vi "Task2.vi"() -> ()   [LabVIEW 2021]
uses:
  <vilib>/myRIO/Instrument Drivers/Utilities/Utilities.lvlib
  <vilib>/Platform/TimedLoop/XDataNode/wakeup.ctl
  <vilib>/Platform/TimedLoop/XDataNode/XDNodeRunTimeDep.lvlib
  <vilib>/Platform/TimedLoop/XDataNode/nitl_modes.ctl
  <vilib>/Platform/TimedLoop/XDataNode/timing_clust.ctl
  <vilib>/Platform/TimedLoop/XDataNode/XDataNode.xnode
  <vilib>/myRIO/Instrument Drivers/Onboard IO/AI/AI.lvlib
  <vilib>/myRIO/Common/Instrument Driver Framework/Utilities/typedefs/Analog Scaling Constants.ctl
  <vilib>/myRIO/Common/Instrument Driver Framework/Utilities/typedefs/Analog Scaling Constants List.ctl
  <vilib>/myRIO/Common/Instrument Driver Framework/myRIO v1.0/AI/typedefs/AI Channels Enum.ctl
  <vilib>/myRIO/Common/Instrument Driver Framework/myRIO v1.0/AI/typedefs/AI Channels List.ctl
  <vilib>/myRIO/Common/Instrument Driver Framework/Utilities/typedefs/Generic FPGA Reference.ctl
  <vilib>/myRIO/Common/Instrument Driver Framework/Utilities/typedefs/myRIO v1.0 Reference.ctl
  <vilib>/myRIO/Common/Instrument Driver Framework/Utilities/typedefs/Hardware Version Enum.ctl
  <vilib>/myRIO/Common/Instrument Driver Framework/Utilities/typedefs/myRIO Generic Hardware Reference.ctl
  <vilib>/myRIO/Instrument Drivers/Onboard IO/AI/typedefs/AI Reference.ctl
  <vilib>/userDefined/High Color/nirio_resource_hc.ctl
  <vilib>/myRIO/Common/Instrument Driver Framework/myRIO v1.0/AI/vis/myRIO v1.1 Open AI.vi
  <vilib>/myRIO/Instrument Drivers/Onboard IO/AI/vis/myRIO AI Open.xnode
panel:
  in  "Stop Button":bool
  in  "Tab Control":enum32{"Noise Exposure", "Custom Graphs"}(tab)
  in  "Graph Time Max":dbl=5.0
  in  "Graph Time Min":dbl
  out "Microphone":waveform(dbl)(graph)
  in  "Seconds to Record":dbl=2.0 min=0.0 step=0.1
  out "Request Exceeds \n100,000 samples":bool
  in  "Collect Data":bool
  out "Acquiring":bool
  out "Pk-Pk":dbl format="%.2p"
  out "RMS":dbl format="%.2p"
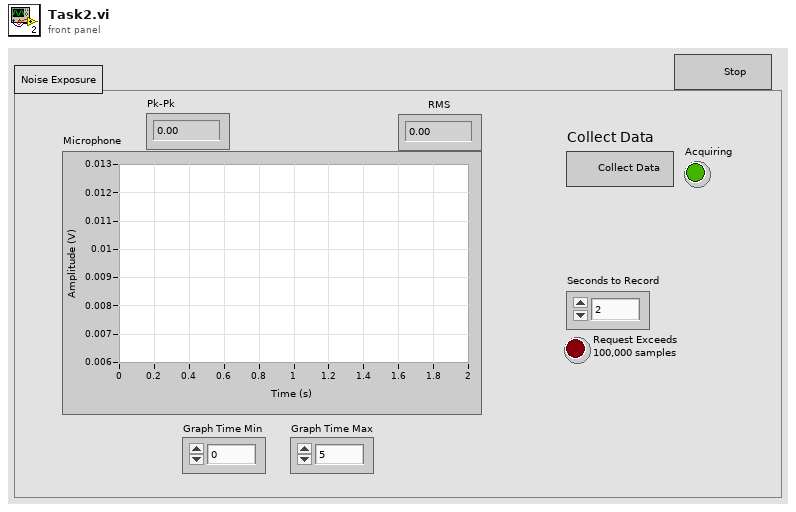
[diagram p1: front panel]
types:
  T1 = typedef "XDNodeRunTimeDep.lvlib/timing_clust.ctl" = cluster{"Expected End [f-1]":u64, "Actual End [f-1]":u64, "Finished Late? [f-1]":bool, "Expected End [i-1]":u64, "Actual End [i-1]":u64, "Finished Late? [i-1]":bool, "Expected Start [i]":u64, "Actual Start [i]":u64, "Expected Start [f]":u64, "Actual Start [f]":u64, "Source Name":string, "Structure Name":string, "Period":i64, "Deadline":i64, "Offset":i64, "Start":i64, "Priority":i32, "Timeout":i32, "Mode":T2, "Wakeup Reason":T3, "Error":errorcluster, "Source Type":string, "Secondary Source Type":string, "Global End Time":u64, "Global Start Time":u64, "Frame Duration":u64, "Iteration Duration":u64, "Assigned CPU":i32, "I/O Scan Engine Mode":u32}
  T2 = typedef "XDNodeRunTimeDep.lvlib/nitl_modes.ctl" = enum32{"No Change", "Process missed periods, maintain original phase", "Discard missed periods, maintain original phase", "Process missed periods, ignore original phase", "Discard missed periods, ignore original phase"}
  T3 = typedef "XDNodeRunTimeDep.lvlib/wakeup.ctl" = enum32{"Normal", "Aborted", "Asynchronous wakeup", "Timing source error", "Timed loop error", "Timeout"}
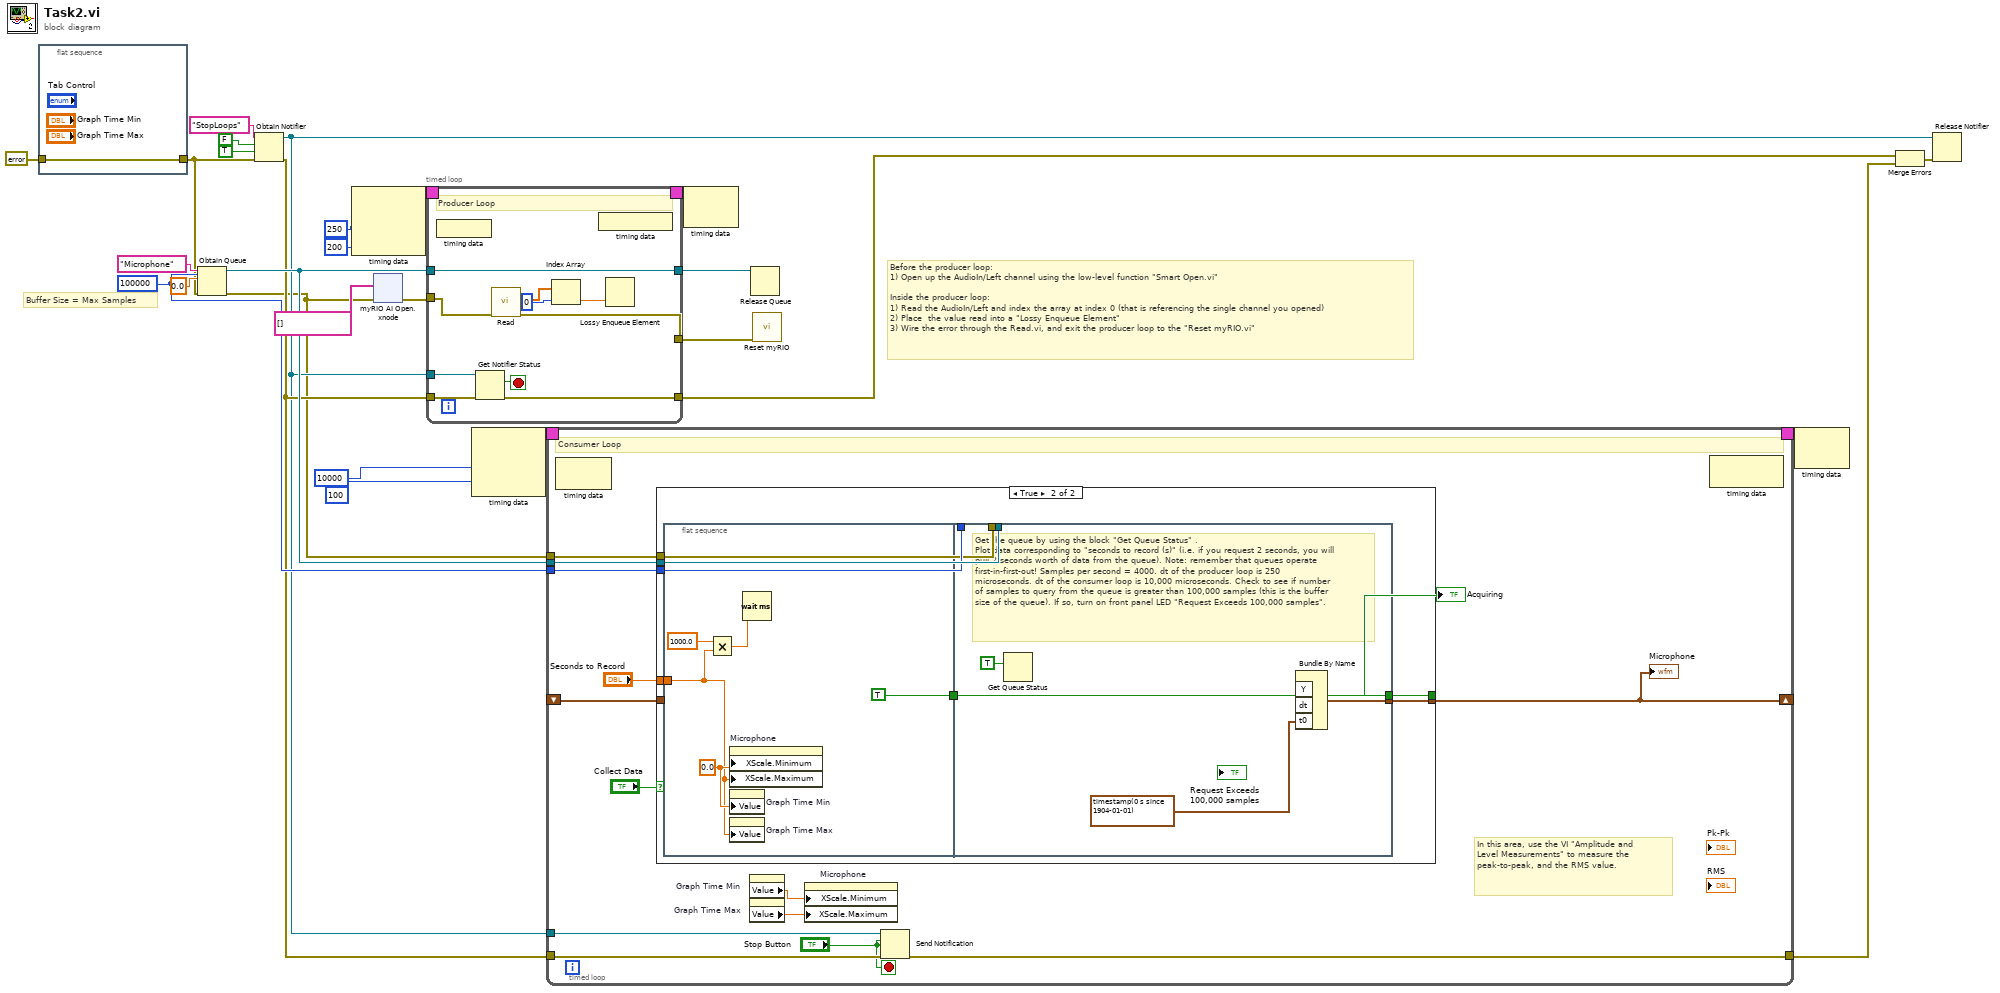
[diagram p0: block diagram]
diagram:
  w9 = 100000 ("max queue size (-1, unlimited)")
  # "Before the producer loop:\n1) Open up the AudioIn/Left channel using the low-level function \"Smart Open.vi\"\n\nInside the producer loop:\n1) Read the AudioIn/Left and index the array at index 0 (that is referencing the single channel you opened)\n2) Place  the value read into a \"Lossy Enqueue Element\"\n3) Wire the error through the Read.vi, and exit the producer loop to the \"Reset myRIO.vi\""
  # "Buffer Size = Max Samples"
  n1 = flat-sequence {
    tunnel: errorcluster {"status"=FALSE, "code"=0, "source"=""} ("error in") -> [w28]
    tunnel: [w28] -> w7
    frame #0 {
    }
  }
  n2 = Obtain Queue(max queue size (-1, unlimited)=w9, name (unnamed)="Microphone", element data type=0.0 ("x-y"), error in (no error)=w7) -> (queue out=w6:refnum<queue>, error out=w2:errorcluster)  [unwired: 1 in, 1 out]
  n3 = Obtain Notifier(name (unnamed)="StopLoops", notification data type=FALSE ("Stop Button"), create if not found? (T)=TRUE, error in (no error)=w7) -> (notifier out=w4:refnum<notifier>, error out=w5:errorcluster)  [unwired: 1 out]
  n4 = node-c288(i64 250 ("Period"), 200 ("Priority")) -> (w27:T1)  [unwired: 1 in]
  n5 = xnode "myRIO AI Open.xnode"("error in (no error)"=w2, "Channel Names"=tag[] []) -> ("error out"=w1:errorcluster)  [unwired: 1 in, 1 out]
  n6 = timed-loop "Timed Loop" {
    timing: w27 -> [_]
    timing-out: [_] -> w26
    tunnel: w1 -> [w33]
    tunnel: [w32] -> w16
    tunnel: w6 -> [w34]
    tunnel: [w34] -> w21
    tunnel: w5 -> [w37]
    tunnel: [w36] -> w13
    tunnel: w4 -> [w38]
    stop <- w35 stop-if-true
    # "Producer Loop"
    n7 = node-c288() -> ()  [unwired: 1 in]
    n8 = Get Notifier Status(notifier=w38, error in (no error)=w37) -> (current notification=w35:bool, error out=w36:errorcluster)  [unwired: 3 out]
    n9 = call <vilib>:"Read.vi"("error in (no error)"=w33) -> ("error out"=w32:errorcluster, "Values"=w31:dbl[])  [unwired: 8 in, 1 out]
    n10 = Index Array(array=w31, index=0) -> (element=w29:dbl)
    n11 = node-c288() -> ()  [unwired: 1 out]
    n12 = Lossy Enqueue Element(element=w29) -> ()  [unwired: 2 in, 4 out]
  }
  n13 = node-c288(i64 10000 ("Period"), 100 ("Priority")) -> (w25:T1)  [unwired: 1 in]
  n14 = timed-loop {
    tunnel: w5 -> [w47]
    tunnel: w4 -> [w48]
    tunnel: [w46] -> w12
    tunnel: w9 -> [w52]
    tunnel: w6 -> [w53]
    shift-right: [w43] -> _
    shift-left: _ -> [w54]
    timing: w25 -> [_]
    timing-out: [_] -> w24
    tunnel: w2 -> [w44]
    stop <- "Stop Button" stop-if-true
    # "In this area, use the VI \"Amplitude and Level Measurements\" to measure the peak-to-peak, and the RMS value."
    # "Consumer Loop"
    n15 = node-c288() -> ()  [unwired: 1 in, 1 out]
    n16 = case shown="True" "Collect Data" {
      tunnel: [w57 w64] -> w43
      tunnel: w54 -> [w57 _]
      tunnel: w53 -> [_ w63]
      tunnel: w52 -> [_ w62]
      tunnel: w44 -> [_ w61]
      tunnel: "Seconds to Record" -> [_ w60]
      tunnel: [_ w59] -> w41
      frame False {
      }
      frame True {
        n17 = flat-sequence {
          tunnel: w60 -> [w68]
          tunnel: [TRUE] -> w58
          tunnel: w62 -> [_]
          tunnel: w63 -> [_]
          tunnel: [w73] -> w64
          tunnel: w61 -> [_]
          tunnel: [w71] -> w59
          tunnel: w58 -> [w71]
          frame #0 {
            w69 = 0.0 ("X Scale.Range:Minimum")
            n18 = Multiply(x=1000.0, y=w68) -> (x*y=w66:dbl)
            n19 = property on="Microphone" class="WFGraph (strict)"("XScale.Minimum"=w69, "XScale.Maximum"=w68) -> ()  [unwired: 2 in, 2 out]
            n20 = property on="Graph Time Min" class="DigNum (strict)"("Value"=w69) -> ()  [unwired: 2 in, 2 out]
            n21 = property on="Graph Time Max" class="DigNum (strict)"("Value"=w68) -> ()  [unwired: 2 in, 2 out]
            n22 = Wait (ms)(milliseconds to wait=w66) -> ()  [unwired: 1 out]
          }
          frame #1 {
            # "Get the queue by using the block \"Get Queue Status\" . \nPlot data corresponding to \"seconds to record (s)\" (i.e. if you request 2 seconds, you will pull 2 seconds worth of data from the queue). Note: remember that queues operate first-in-first-out! Samples per second = 4000. dt of the producer loop is 250 microseconds. dt of the consumer loop is 10,000 microseconds. Check to see if number of samples to query from the queue is greater than 100,000 samples (this is the buffer size of the queue). If so, turn on front panel LED \"Request Exceeds 100,000 samples\"."
            n23 = Get Queue Status(return elements? (F)=TRUE) -> ()  [unwired: 2 in, 8 out]
            n24 = Bundle By Name("t0"=timestamp(0 s since 1904-01-01)) -> (w73:waveform(dbl))  [unwired: 3 in]
          }
        }
      }
    }
    "Microphone" <- w43
    "Acquiring" <- w41
    n25 = property on="Graph Time Min" class="DigNum (strict)"() -> ("Value"=w49:dbl)  [unwired: 2 in, 2 out]
    n26 = property on="Graph Time Max" class="DigNum (strict)"() -> ("Value"=w50:dbl)  [unwired: 2 in, 2 out]
    n27 = property on="Microphone" class="WFGraph (strict)"("XScale.Minimum"=w49, "XScale.Maximum"=w50) -> ()  [unwired: 2 in, 2 out]
    n28 = Send Notification(notification="Stop Button", notifier=w48, error in (no error)=w47) -> (error out=w46:errorcluster)  [unwired: 1 out]
    n29 = node-c288() -> ()  [unwired: 1 in, 1 out]
  }
  n30 = node-c288(w26) -> ()  [unwired: 1 out]
  n31 = Release Queue(queue=w21) -> ()  [unwired: 2 in, 3 out]
  n32 = call <vilib>:"Reset myRIO.vi"("error in (no error)"=w16) -> ()  [unwired: 10 in, 1 out]
  n33 = node-c288(w24) -> ()  [unwired: 1 out]
  n34 = Merge Errors(w13, w12) -> (w17:errorcluster)
  n35 = Release Notifier(notifier=w4, error in (no error)=w17) -> ()  [unwired: 1 in, 3 out]
